vi "PAM Parse Header.vi"(0 "icListen #":i32, 1 "Header":string) -> (14 "Timestamp":u64)   [LabVIEW 2020]
uses:
  PAM Volts per Bit.vi
  PAM uPa per Volts.vi
  PAM uPa per Bit.vi
  icListen 1 Metadata.vi
  icListen 2 Metadata.vi
  icListen 3 Metadata.vi
  icListen 4 Metadata.vi
  PAM Library.lvlib
panel:
  out "Instrument Time":string
  out "Instrument Date":string
  out "Sample Number":u32
  out "uPa per Volts":dbl
  out "Volts per Bit":dbl
  out "Bytes Per Sample":u32
  out "uPa per Bit":dbl
  out "Payload Length":string
  out "Chunk Size":u16
  out "Number of Samples":u16
  out "Data":string
  out "Data Chunk Header":string
  out "Event Key":string
  out "Type, Sync":string
  out "Payload Length":u8
  out "Data Scale":T1 {"Sensitivity" format="%#_4g"}
  out "Data Format":T2
  out "Metadata":T3 {"Temperature" format="%#_3g"; "Humidity" format="%_3f"}
  out "Min Count":i32
  out "Unit of Measure":u8
  out "Little Endian?":bool
  out "Sensitivity":dbl format="%_4f"
  out "Serial Number":u16
  out "Battery Charge":u8
  out "Humidity":dbl format="%_3f"
  out "Temperature":dbl format="%_3f"
  out "Max Count":i32
  out "Min Amplitude":i32
  out "Max Amplitude":i32
  out "Channel #":u8
  out "Gain":i32
  out "Sample Rate":i32
  out "Date":string
  out "Time":string
  out "Amplitude Scaling":string
  out "Setup":string
  out "Status":string
  out "Device Info":string
  out "Event Key":string
  out "Type, Sync":string
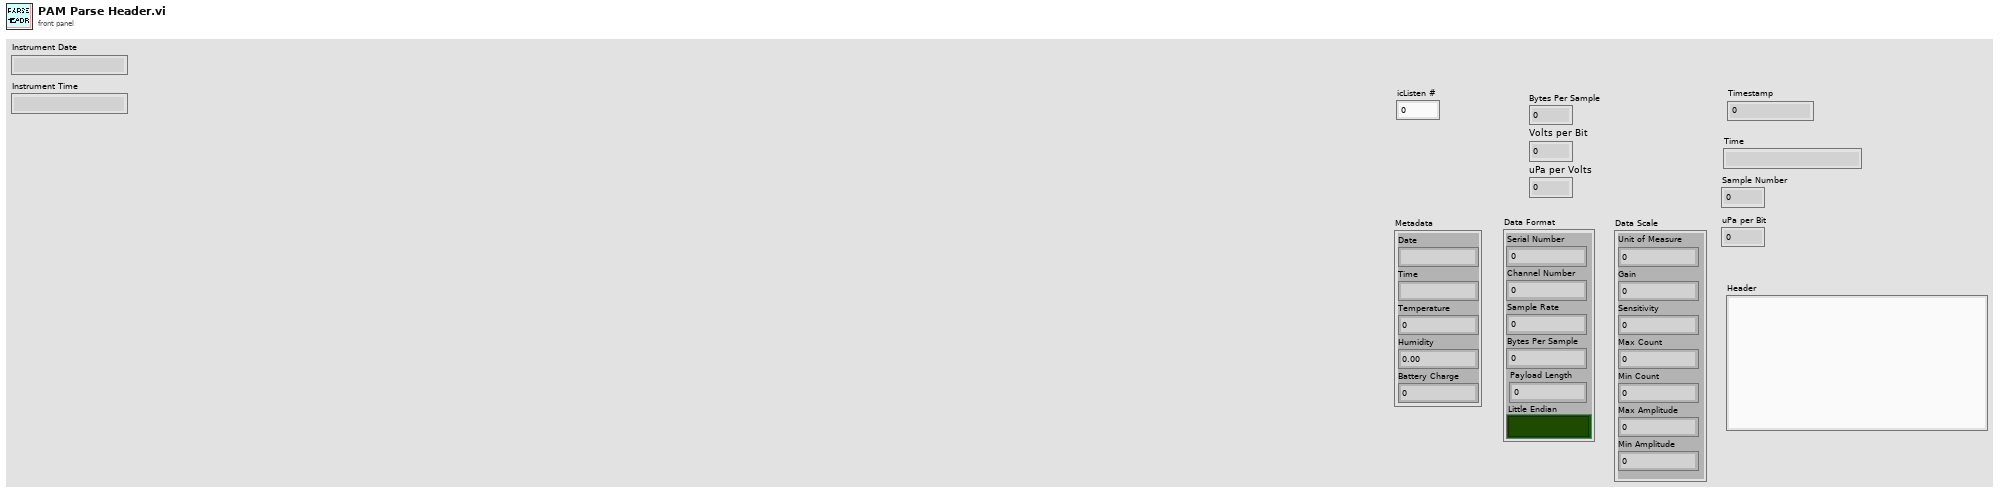
[diagram p1: front panel]
types:
  T1 = cluster{"Unit of Measure":u8, "Gain":i32, "Sensitivity":dbl, "Max Count":i32, "Min Count":i32, "Max Amplitude":i32, "Min Amplitude":i32}
  T2 = cluster{"Serial Number":i32, "Channel Number":u8, "Sample Rate":i32, "Bytes Per Sample":u32, "Payload Length":dbl, "Little Endian":bool}
  T3 = cluster{"Date":string, "Time":string, "Temperature":dbl, "Humidity":dbl, "Battery Charge":i32}
  T4 = cluster{"date string":string, "time string":string, dbl, dbl, u8}
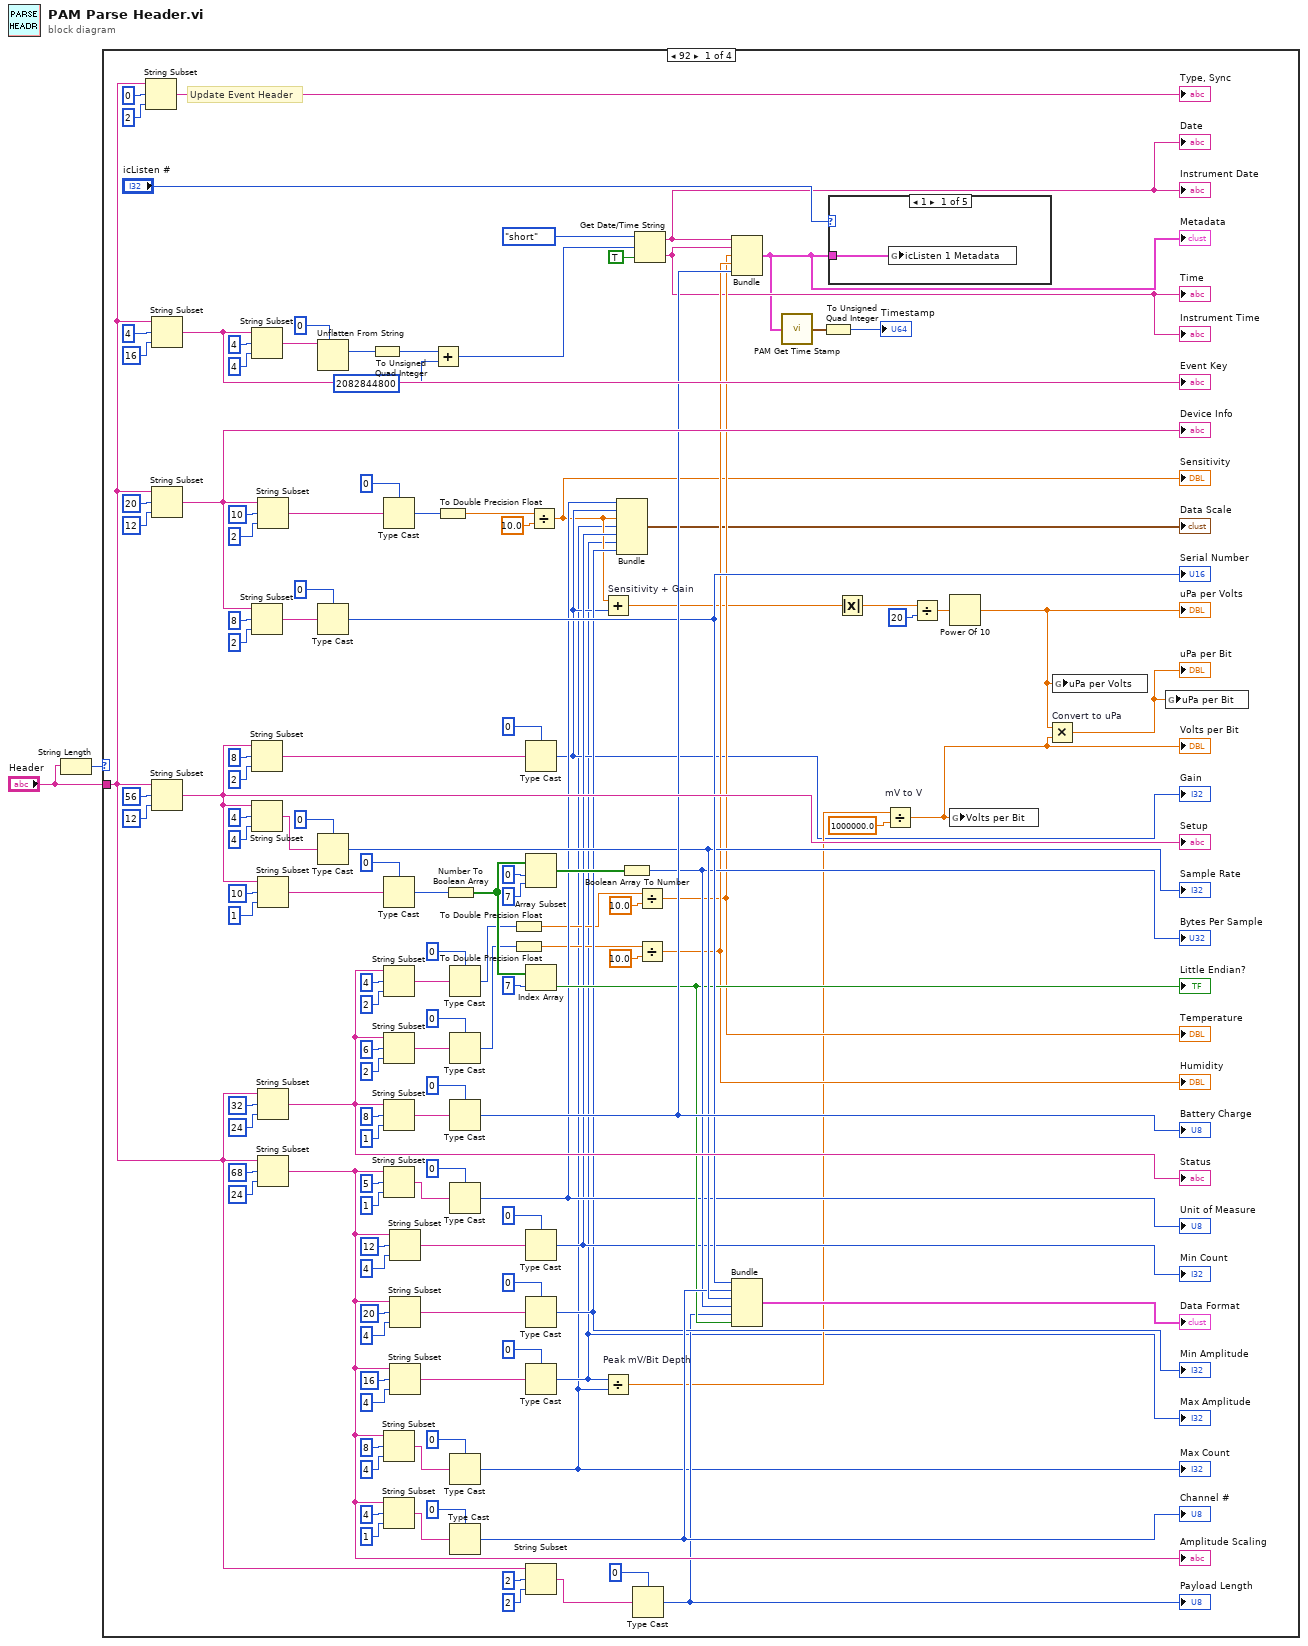
[diagram p0: block diagram]
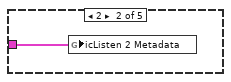
[diagram p2: hidden frame]
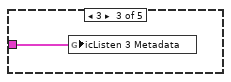
[diagram p3: hidden frame]
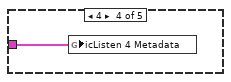
[diagram p4: hidden frame]
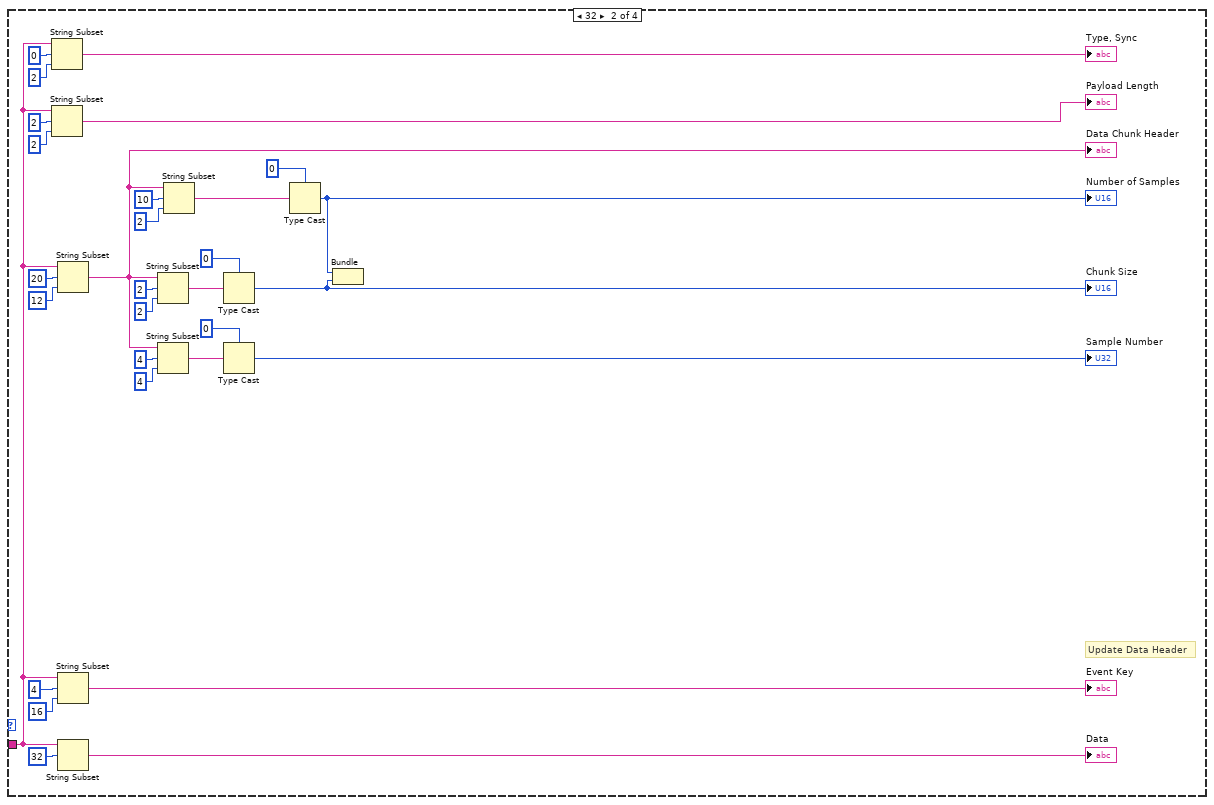
[diagram p6: hidden frame]
diagram:
  n1 = String Length(string="Header") -> (length=w2:i32)
  n2 = case shown="92" w2 {
    tunnel: "Header" -> [w31 w149 _ _]
    frame 92 {
      # "Update Event Header"
      n3 = String Subset(string=w31, offset (0)=0, length (rest)=2 ("length (rest)")) -> (substring=→"Type, Sync":string)
      n4 = String Subset(string=w31, offset (0)=4, length (rest)=16 ("length (rest)")) -> (substring=w127:string)
      "Event Key" <- w127
      n5 = String Subset(string=w31, offset (0)=20, length (rest)=12 ("length (rest)")) -> (substring=w78:string)
      "Device Info" <- w78
      n6 = String Subset(string=w31, offset (0)=56, length (rest)=12 ("length (rest)")) -> (substring=w67:string)
      "Setup" <- w67
      n7 = String Subset(string=w127, offset (0)=4, length (rest)=4 ("length (rest)")) -> (substring=w6:string)
      n8 = String Subset(string=w78, offset (0)=8, length (rest)=2 ("length (rest)")) -> (substring=w84:string)
      n9 = String Subset(string=w67, offset (0)=8, length (rest)=2 ("length (rest)")) -> (substring=w112:string)
      n10 = String Subset(string=w67, offset (0)=4, length (rest)=4 ("length (rest)")) -> (substring=w114:string)
      n11 = String Subset(string=w78, offset (0)=10, length (rest)=2 ("length (rest)")) -> (substring=w80:string)
      n12 = String Subset(string=w67, offset (0)=10, length (rest)=1 ("length (rest)")) -> (substring=w75:string)
      n13 = String Subset(string=w31, offset (0)=32, length (rest)=24 ("length (rest)")) -> (substring=w87:string)
      "Status" <- w87
      n14 = String Subset(string=w31, offset (0)=68, length (rest)=24 ("length (rest)")) -> (substring=w58:string)
      "Amplitude Scaling" <- w58
      n15 = Unflatten From String(type=u32 0, binary string=w6) -> (value=w9:u32)  [unwired: 3 in, 2 out]
      n16 = Type Cast(type=u16 0, x=w84) -> (*(type *) &x=w56:u16)
      "Serial Number" <- w56
      n17 = Type Cast(type=0, x=w114) -> (*(type *) &x=w55:i32)
      "Sample Rate" <- w55
      n18 = To Unsigned Quad Integer(1:w9) -> (0:w11:u64)
      n19 = Type Cast(type=i16 0, x=w80) -> (*(type *) &x=w32:i16)
      n20 = Type Cast(type=u8 0, x=w75) -> (*(type *) &x=w73:u8)
      n21 = String Subset(string=w87, offset (0)=4, length (rest)=2 ("length (rest)")) -> (substring=w97:string)
      n22 = String Subset(string=w87, offset (0)=6, length (rest)=2 ("length (rest)")) -> (substring=w93:string)
      n23 = String Subset(string=w87, offset (0)=8, length (rest)=1 ("length (rest)")) -> (substring=w89:string)
      n24 = String Subset(string=w58, offset (0)=5, length (rest)=1 ("length (rest)")) -> (substring=w63:string)
      n25 = String Subset(string=w58, offset (0)=8, length (rest)=4 ("length (rest)")) -> (substring=w101:string)
      n26 = String Subset(string=w58, offset (0)=4, length (rest)=1 ("length (rest)")) -> (substring=w109:string)
      n27 = String Subset(string=w58, offset (0)=12, length (rest)=4 ("length (rest)")) -> (substring=w59:string)
      n28 = String Subset(string=w58, offset (0)=20, length (rest)=4 ("length (rest)")) -> (substring=w105:string)
      n29 = String Subset(string=w58, offset (0)=16, length (rest)=4 ("length (rest)")) -> (substring=w107:string)
      n30 = Add(x=w11, y=u64 2082844800) -> (x+y=w13:u64)
      n31 = To Double Precision Float(number=w32) -> (double precision float=w33:dbl)
      n32 = Number To Boolean Array(number=w73) -> (Boolean array=w71:bool[])
      n33 = Type Cast(type=i16 0, x=w97) -> (*(type *) &x=w42:i16)
      n34 = Type Cast(type=i16 0, x=w93) -> (*(type *) &x=w46:i16)
      n35 = Type Cast(type=u8 0, x=w89) -> (*(type *) &x=w57:u8)
      "Battery Charge" <- w57
      n36 = Type Cast(type=u8 0, x=w63) -> (*(type *) &x=w51:u8)
      "Unit of Measure" <- w51
      n37 = Type Cast(type=0, x=w101) -> (*(type *) &x=w18:i32)
      "Max Count" <- w18
      n38 = Type Cast(type=u8 0, x=w109) -> (*(type *) &x=w54:u8)
      "Channel #" <- w54
      n39 = To Double Precision Float(number=w42) -> (double precision float=w43:dbl)
      n40 = To Double Precision Float(number=w46) -> (double precision float=w45:dbl)
      n41 = Type Cast(type=0, x=w112) -> (*(type *) &x=w21:i32)
      "Gain" <- w21
      n42 = Array Subset(array=w71, index=0, length=7) -> (w68:bool[])
      n43 = Index Array(array=w71, index=u8 7) -> (element=w52:bool)
      "Little Endian?" <- w52
      n44 = Type Cast(type=0, x=w59) -> (*(type *) &x=w50:i32)
      "Min Count" <- w50
      n45 = Type Cast(type=0, x=w105) -> (*(type *) &x=w49:i32)
      "Min Amplitude" <- w49
      n46 = Type Cast(type=0, x=w107) -> (*(type *) &x=w19:i32)
      "Max Amplitude" <- w19
      n47 = String Subset(string=w31, offset (0)=2, length (rest)=2 ("length (rest)")) -> (substring=w37:string)
      n48 = Divide(x=w33, y=10.0) -> (x/y=w20:dbl)
      "Sensitivity" <- w20
      n49 = Add "Sensitivity + Gain"(x=w20, y=w21) -> (x+y=w28:dbl)
      n50 = Divide "Peak mV/Bit Depth"(x=w19, y=w18) -> (x/y=w25:dbl)
      n51 = Bundle(w51, w21, w20, w18, w50, w19, w49) -> (→"Data Scale":cluster{u8, i32, dbl, i32, i32, i32, i32})  [unwired: 1 in]
      n52 = Boolean Array To Number(Boolean array=w68) -> (number=w53:u32)
      "Bytes Per Sample" <- w53
      n53 = Type Cast(type=u8 0, x=w37) -> (*(type *) &x=w36:u8)
      "Payload Length" <- w36
      n54 = Get Date/Time String(date format (0)=enum16{"short", "long", "abbreviated"}."short", seconds (now)=w13, want seconds? (F)=TRUE) -> (date string=w8:string, time string=w7:string)
      "Time" <- w7
      "Date" <- w8
      "Instrument Date" <- w8
      "Instrument Time" <- w7
      n55 = Divide(x=w43, y=10.0) -> (x/y=w41:dbl)
      "Temperature" <- w41
      n56 = Divide(x=w45, y=10.0) -> (x/y=w47:dbl)
      "Humidity" <- w47
      n57 = Bundle("date string"=w8, "time string"=w7, w41, w47, w57) -> (w5:T4)  [unwired: 1 in]
      "Metadata" <- w5
      n58 = Bundle(w56, w54, w55, w53, w36, w52) -> (→"Data Format":cluster{u16, u8, i32, u32, u8, bool})  [unwired: 1 in]
      n59 = call "PAM Get Time Stamp.vi"("icListen Metadata"=w5) -> ("Time Stamp"=w4:timestamp)
      n60 = To Unsigned Quad Integer(1:w4) -> (0:→"Timestamp":u64)
      n61 = case shown="1" "icListen #" {
        tunnel: w5 -> [w140 w141 w142 w143 _]
        frame 1 {
          n62 = global write "icListen 1 Metadata.vi" "icListen 1 Metadata"(w140) -> ()
        }
        frame 2 {
          n63 = global write "icListen 2 Metadata.vi" "icListen 2 Metadata"(w141) -> ()
        }
        frame 3 {
          n64 = global write "icListen 3 Metadata.vi" "icListen 3 Metadata"(w142) -> ()
        }
        frame 4 {
          n65 = global write "icListen 4 Metadata.vi" "icListen 4 Metadata"(w143) -> ()
        }
        frame 5, Default {
        }
      }
      n66 = Absolute Value(x=w28) -> (abs(x)=w29:dbl)
      n67 = Divide "mV to V"(x=w25, y=1000000.0) -> (x/y=w23:dbl)
      "Volts per Bit" <- w23
      n68 = Divide(x=w29, y=20) -> (x/y=w27:dbl)
      n69 = Power Of 10(x=w27) -> (10^x=w22:dbl)
      "uPa per Volts" <- w22
      n70 = global write "PAM Volts per Bit.vi" "Volts per Bit"(w23) -> ()
      n71 = Multiply "Convert to uPa"(x=w22, y=w23) -> (x*y=w16:dbl)
      "uPa per Bit" <- w16
      n72 = global write "PAM uPa per Volts.vi" "uPa per Volts"(w22) -> ()
      n73 = global write "PAM uPa per Bit.vi" "uPa per Bit"(w16) -> ()
    }
    frame 32 {
      # "Update Data Header"
      n74 = String Subset(string=w149, offset (0)=0, length (rest)=2 ("length (rest)")) -> (substring=→"Type, Sync":string)
      n75 = String Subset(string=w149, offset (0)=2, length (rest)=2 ("length (rest)")) -> (substring=→"Payload Length":string)
      n76 = String Subset(string=w149, offset (0)=20, length (rest)=12 ("length (rest)")) -> (substring=w148:string)
      "Data Chunk Header" <- w148
      n77 = String Subset(string=w149, offset (0)=4, length (rest)=16 ("length (rest)")) -> (substring=→"Event Key":string)
      n78 = String Subset(string=w149, offset (0)=32) -> (substring=→"Data":string)  [unwired: 1 in]
      n79 = String Subset(string=w148, offset (0)=2, length (rest)=2 ("length (rest)")) -> (substring=w157:string)
      n80 = String Subset(string=w148, offset (0)=4, length (rest)=4 ("length (rest)")) -> (substring=w146:string)
      n81 = String Subset(string=w148, offset (0)=10, length (rest)=2 ("length (rest)")) -> (substring=w159:string)
      n82 = Type Cast(type=u16 0, x=w157) -> (*(type *) &x=w151:u16)
      "Chunk Size" <- w151
      n83 = Type Cast(type=u32 0, x=w146) -> (*(type *) &x=→"Sample Number":u32)
      n84 = Type Cast(type=u16 0, x=w159) -> (*(type *) &x=w152:u16)
      "Number of Samples" <- w152
      n85 = Bundle(w152, w151) -> ()  [unwired: 1 in, 1 out]
    }
    frame 8 {
      # "Notification"
    }
    frame 0, Default {
      # "No Header"
    }
  }
